vi "Encoderausgabe.vi"(8 "error in (no error)":errorcluster, 11 "Reset":bool) -> (0 "error out":errorcluster, 3 "Numeric":dbl)   [LabVIEW 2018]
doc: "The myRIO Project template acquires acceleration data from the onboard accelerometer and displays the changes of acceleration values in a waveform chart."
uses:
  <vilib>/myRIO/Common/Instrument Driver Framework/Utilities/typedefs/Generic FPGA Reference.ctl
  <vilib>/myRIO/Common/Instrument Driver Framework/Utilities/typedefs/myRIO v1.0 Reference.ctl
  <vilib>/myRIO/Common/Instrument Driver Framework/Utilities/typedefs/Hardware Version Enum.ctl
  <vilib>/myRIO/Common/Instrument Driver Framework/Utilities/typedefs/myRIO Generic Hardware Reference.ctl
  <vilib>/myRIO/Common/Instrument Driver Framework/myRIO v1.0/Encoder/typedefs/Encoder Channels Enum.ctl
  <vilib>/myRIO/Instrument Drivers/Onboard IO/Encoder/typedefs/Encoder Reference.ctl
  <vilib>/myRIO/Instrument Drivers/Onboard IO/Encoder/Encoder.lvlib
  <vilib>/myRIO/Common/Instrument Driver Framework/myRIO v1.0/Encoder/typedefs/Encoder Signal Mode.ctl
  <vilib>/myRIO/Instrument Drivers/Onboard IO/Encoder/vis/myRIO Encoder Open.xnode
  <vilib>/myRIO/Common/Instrument Driver Framework/myRIO v1.0/Encoder/vis/myRIO v1.1 Open Encoder.vi
  <vilib>/myRIO/Common/Instrument Driver Framework/myRIO v1.0/Encoder/vis/myRIO v1.0 Configure Encoder.vi
  <vilib>/myRIO/Common/Instrument Driver Framework/myRIO v1.0/Encoder/typedefs/Encoder Configuration v1.0.ctl
  <vilib>/userdefined/High Color/nirio_resource_hc.ctl
panel:
  out "Waveform Chart 2":i32(graph)
  in  "stop":bool
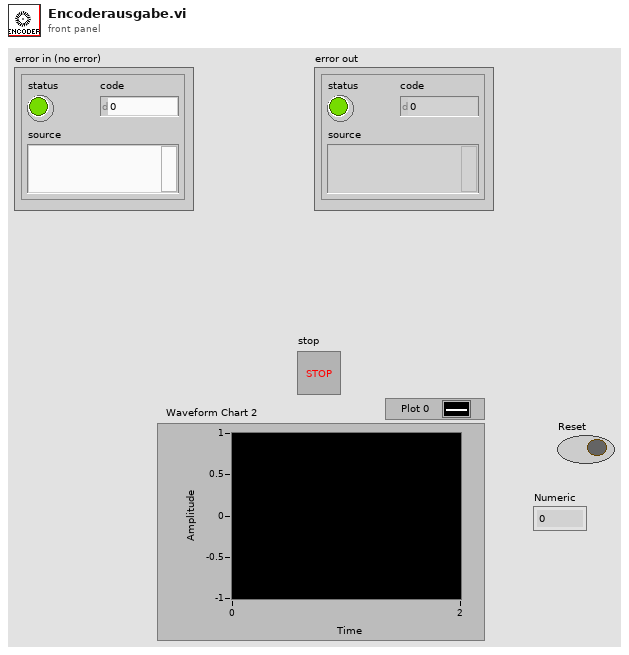
[diagram p1: front panel]
types:
  T1 = typedef "Encoder.lvlib/Encoder Reference.ctl" = cluster{"myRIO Reference":T2, "Encoder Channels Enum":T6}
  T2 = typedef "myRIO Generic Hardware Reference.ctl" = cluster{"myRIO Model":T3, "myRIO Hardware Reference":T4}
  T3 = typedef "Hardware Version Enum.ctl" = enum16{"Unknown", "myRIO-1900", "myRIO-1950", "roboRIO", "NI ELVIS RIO CM", "ELVIS III"}
  T4 = typedef "myRIO v1.0 Reference.ctl" = cluster{"Generic FPGA Reference":T5, "Allow multiple opens":bool}
  T5 = typedef "Generic FPGA Reference.ctl" = refnum<k20>
  T6 = typedef "Encoder Channels Enum.ctl" = enum16{"Not Connected", "C/ENC0", "C/ENC1", "A/ENC", "A/ENC0", "A/ENC1", "A/ENC2", "A/ENC3", "A/ENC4", "A/ENC5", "A/ENC6", "A/ENC7", "A/ENC8", "A/ENC9", "B/ENC", "B/ENC0", "B/ENC1", "B/ENC2", "B/ENC3", "B/ENC4", "B/ENC5", "B/ENC6", "B/ENC7", "B/ENC8", "B/ENC9", "DIO/ENC0", "DIO/ENC1", "DIO/ENC2", "DIO/ENC3", "DIO/ENC4"}
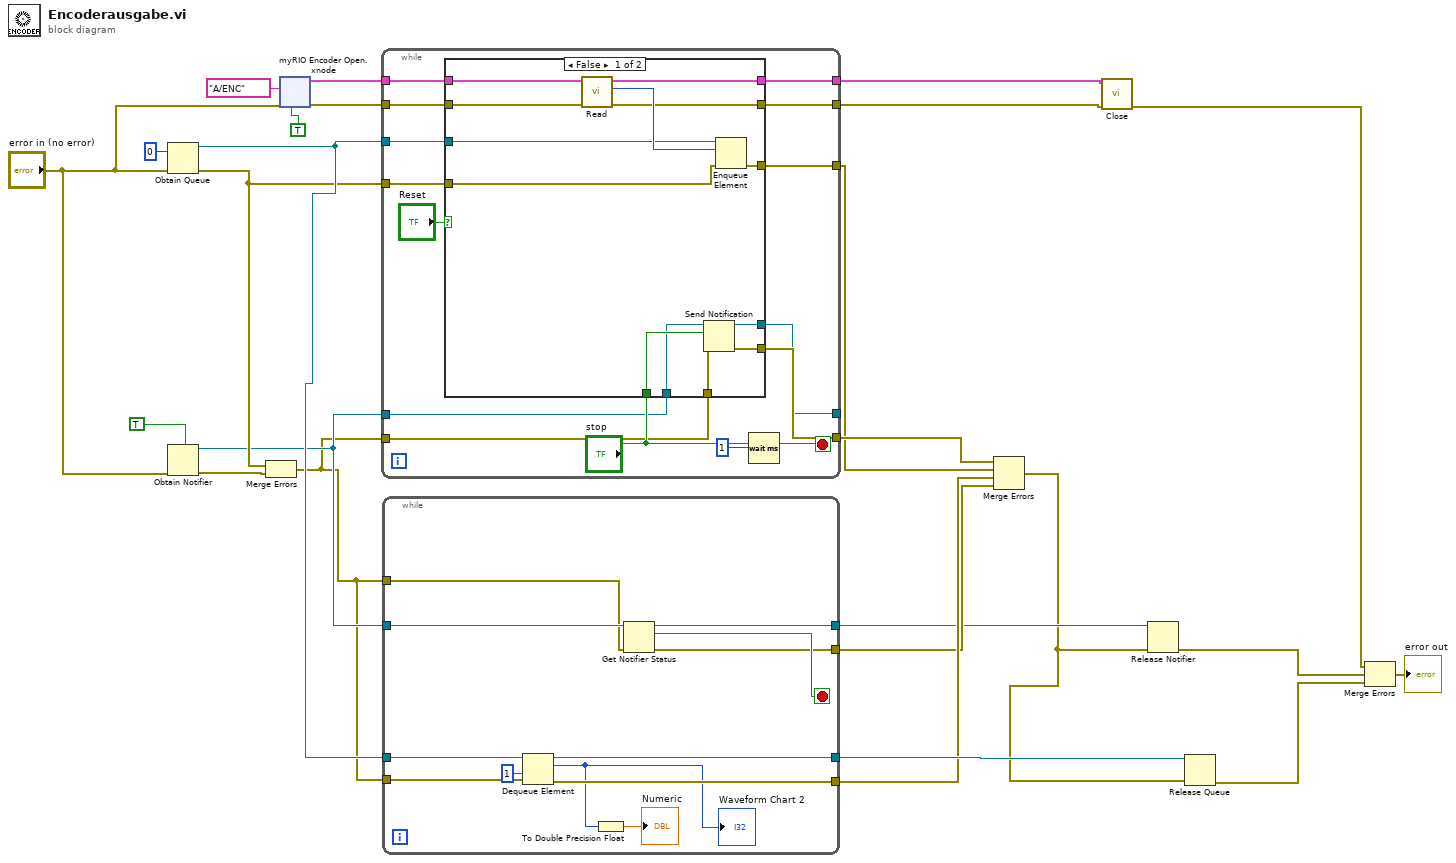
[diagram p0: block diagram]
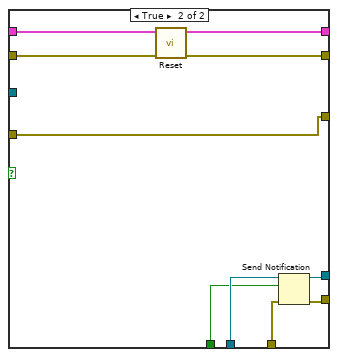
[diagram p2: hidden frame]
diagram:
  n1 = Obtain Queue(element data type=0 ("Counter Value"), error in (no error)="error in (no error)") -> (queue out=w23:refnum<queue>, error out=w20:errorcluster)  [unwired: 3 in, 1 out]
  n2 = Obtain Notifier(notification data type=TRUE, error in (no error)="error in (no error)") -> (notifier out=w17:refnum<notifier>, error out=w15:errorcluster)  [unwired: 2 in, 1 out]
  n3 = Merge Errors(w20, w15) -> (w14:errorcluster)
  n4 = xnode "myRIO Encoder Open.xnode"("error in (no error)"="error in (no error)", "Channel Name"=tag "A/ENC", "Start Counter"=TRUE) -> ("error out"=w4:errorcluster, "Encoder Ref Out"=w24:T1)  [unwired: 2 in]
  n5 = while {
    tunnel: w24 -> [w38]
    tunnel: w23 -> [w37]
    tunnel: w20 -> [w36]
    tunnel: [w35] -> w7
    tunnel: w17 -> [w33]
    tunnel: w14 -> [w32]
    tunnel: [w31] -> w13
    tunnel: [w30] -> _
    tunnel: w4 -> [w29]
    tunnel: [w28] -> w3
    tunnel: [w27] -> w1
    stop <- "stop" stop-if-true
    n6 = case shown="False" "Reset" {
      tunnel: w38 -> [w52 w62]
      tunnel: w37 -> [w50 _]
      tunnel: w36 -> [w49 w58]
      tunnel: [w48 w58] -> w35
      tunnel: "stop" -> [w47 w53]
      tunnel: w33 -> [w46 w57]
      tunnel: w32 -> [w45 w54]
      tunnel: [w44 w55] -> w31
      tunnel: [w43 w56] -> w30
      tunnel: w29 -> [w42 w60]
      tunnel: [w41 w59] -> w28
      tunnel: [w40 w61] -> w27
      frame False {
        n7 = call <vilib>:"Read.vi"("error in (no error)"=w42, "Encoder Ref In"=w52) -> ("error out"=w41:errorcluster, "Counter Value"=w51:i32, "Encoder Ref Out"=w40:T1)  [unwired: 5 in, 2 out]
        n8 = Send Notification(notification=w47, notifier=w46, error in (no error)=w45) -> (notifier out=w43:refnum<notifier>, error out=w44:errorcluster)
        n9 = Enqueue Element(queue=w50, element=w51, error in (no error)=w49) -> (error out=w48:errorcluster)  [unwired: 1 in, 2 out]
      }
      frame True {
        n10 = call <vilib>:"Reset.vi"("error in (no error)"=w60, "Encoder Ref In"=w62) -> ("error out"=w59:errorcluster, "Encoder Ref Out"=w61:T1)  [unwired: 8 in]
        n11 = Send Notification(notification=w53, notifier=w57, error in (no error)=w54) -> (notifier out=w56:refnum<notifier>, error out=w55:errorcluster)
      }
    }
    n12 = Wait (ms)(milliseconds to wait=u32 1) -> ()  [unwired: 1 out]
  }
  n13 = while {
    tunnel: w14 -> [w68]
    tunnel: w23 -> [w74]
    tunnel: [w73] -> w21
    tunnel: w14 -> [w72]
    tunnel: [w71] -> w16
    tunnel: w17 -> [w69]
    tunnel: [w67] -> w12
    tunnel: [w66] -> w11
    stop <- w70 stop-if-true
    n14 = Dequeue Element(queue=w74, timeout in ms (-1)=1, error in (no error)=w72) -> (queue out=w73:refnum<queue>, element=w63:i32, error out=w71:errorcluster)  [unwired: 1 out]
    "Waveform Chart 2" <- w63
    n15 = To Double Precision Float(number=w63) -> (double precision float=→"Numeric":dbl)
    n16 = Get Notifier Status(notifier=w69, error in (no error)=w68) -> (notifier out=w66:refnum<notifier>, current notification=w70:bool, error out=w67:errorcluster)  [unwired: 2 out]
  }
  n17 = Merge Errors(w13, w7, w16, w12) -> (w10:errorcluster)
  n18 = call <vilib>:"Close.vi"("error in (no error)"=w3, "Encoder Ref In"=w1) -> ("error out"=w6:errorcluster)  [unwired: 9 in]
  n19 = Release Notifier(notifier=w11, error in (no error)=w10) -> (error out=w9:errorcluster)  [unwired: 1 in, 2 out]
  n20 = Release Queue(queue=w21, error in (no error)=w10) -> (error out=w8:errorcluster)  [unwired: 1 in, 2 out]
  n21 = Merge Errors(w6, w9, w8) -> (→"error out":errorcluster)
